vi "Dpc Get Reg Repeat.vi"(0 "hif":u32, 1 "perc":i32, 5 "bAddr":u8, 7 "rgbData":string, 9 "cbData":i32, 11 "error in (no error)":errorcluster, 12 "ptrid":u16) -> (3 "perc out":i32, 4 "hif out":u32, 6 "function return":i32, 8 "rgbData out":string, 14 "ptrid out":u16, 15 "error out":errorcluster)   [LabVIEW 2011, in "LVH-Adept.lvlib" / "DPCUTIL.lvlib"]
doc: "DPCAPI BOOL DpcGetRegRepeat(HANDLE hif, BYTE bAddr, BYTE * rgbData, INT32 cbData, ERC * perc, TRID * ptrid);"
uses:
  DPCUTIL.lvlib
  dpcutil.dll
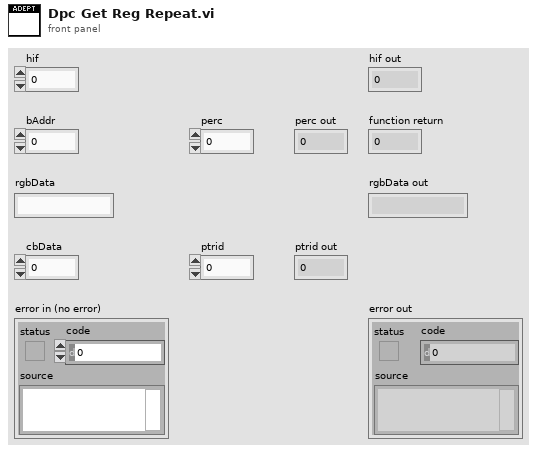
[diagram p1: front panel]
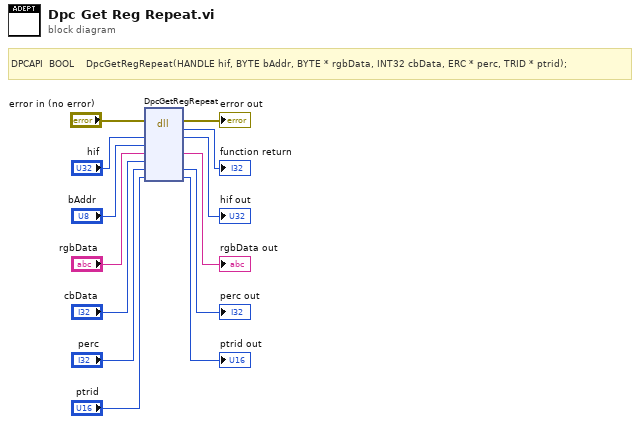
[diagram p0: block diagram]
diagram:
  # "DPCAPI  BOOL    DpcGetRegRepeat(HANDLE hif, BYTE bAddr, BYTE * rgbData, INT32 cbData, ERC * perc, TRID * ptrid);"
  n1 = dll-call lib="dpcutil.*" fn="DpcGetRegRepeat"(error in="error in (no error)", "hif"="hif", "bAddr"="bAddr", "rgbData"="rgbData", "cbData"="cbData", "perc"="perc", "ptrid"="ptrid") -> (error out=→"error out":errorcluster, →"function return":i32, "hif"=→"hif out":u32, "rgbData"=→"rgbData out":string, "perc"=→"perc out":i32, "ptrid"=→"ptrid out":u16)  [unwired: 4 in, 1 out]
